vi "Material Data Extractor.vi"(8 "Error In":errorcluster, 9 "Material Data":variant[][](array[variant])=[[variant]], 10 "Material Name":string, 11 "Ratio":dbl) -> (0 "Error Out":errorcluster, 2 "Exists?":bool, 3 "Material Information":T1)   [LabVIEW 2020]
uses:
  <vilib>/addons/database/_DB Variant To Data/Database Variant To Data.xnode
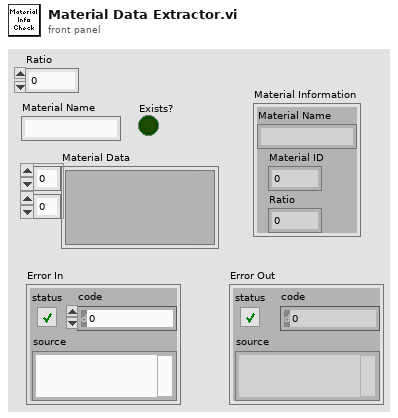
[diagram p1: front panel]
types:
  T1 = cluster{"Material Name":string, "Material ID":i32, "Ratio":dbl}
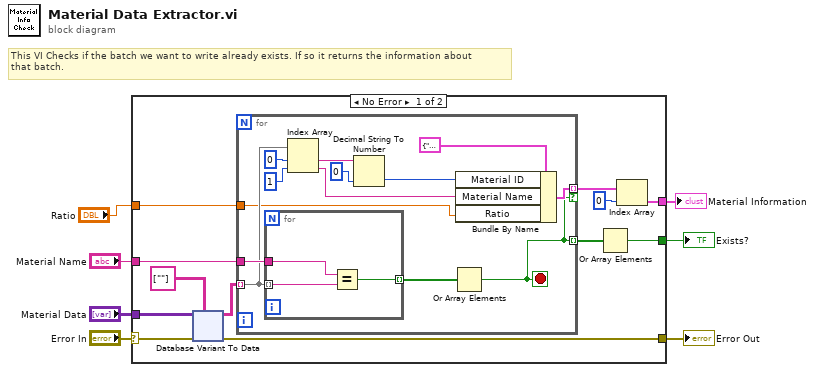
[diagram p0: block diagram]
diagram:
  # "This VI Checks if the batch we want to write already exists. If so it returns the information about\nthat batch."
  n1 = case shown="No Error" "Error In" {
    selector: "Error In" -> [w15 w80]
    tunnel: "Material Data" -> [w16 _]
    tunnel: "Material Name" -> [w14 _]
    tunnel: [w12 _] -> w4
    tunnel: [w13 w80] -> w3
    tunnel: [w9 _] -> w1
    tunnel: "Ratio" -> [w8 _]
    frame No Error {
      n2 = xnode "Database Variant To Data"("database variant"=w16, "error in (no error)"=w15, "type"=string[][] [[""]] ("columns")) -> ("data"=w17:string[][], "error out"=w13:errorcluster)
      n3 = for {
        tunnel: w17 -> [w22] mode=indexing
        tunnel: w14 -> [w32]
        tunnel: [w21] -> w18 mode=indexing
        tunnel: [w23] -> w11 mode=indexing if=w21
        tunnel: w8 -> [w20]
        stop <- w21 stop-if-true
        n4 = for {
          tunnel: w22 -> [w34] mode=indexing
          tunnel: w32 -> [w35]
          tunnel: [w33] -> w31 mode=indexing
          n5 = Equal?(x=w35, y=w34) -> (x = y?=w33:bool)
        }
        n6 = Index Array(array=w22, index #1=0 ("index"), index #2=1 ("index")) -> (element #1=w28:string, element #2=w25:string)
        n7 = Decimal String To Number(string=w28, default (0L)=0 ("default (0 I32)")) -> (number=w24:i32)  [unwired: 1 in, 1 out]
        n8 = Or Array Elements(Boolean array=w31) -> (logical OR=w21:bool)
        n9 = Bundle By Name(cluster=T1 {"Material Name"="", "Material ID"=0, "Ratio"=0.0} ("output cluster"), "Material ID"=w24, "Material Name"=w25, "Ratio"=w20) -> (w23:T1)
      }
      n10 = Or Array Elements(Boolean array=w18) -> (logical OR=w12:bool)
      n11 = Index Array(array=w11, index=0) -> (element=w9:T1)
    }
    frame Error {
    }
  }
  "Exists?" <- w4
  "Error Out" <- w3
  "Material Information" <- w1
